vi "read Aux3 from daq 2016.vi"(4 "Descriptions":string[](array[string]), 5 "error in (no error)":errorcluster, 6 "Aux 3 Slope":dbl=1.7339999675750732 format="%.2f", 10 "Array in":refnum<k24>[](array[refnum]), 11 "Sensor Cluster In":T1) -> (12 "Array out":refnum<k24>[](array[refnum]), 13 "Sensor Cluster 2":T1, 14 "Aux3/EC":dbl format="%.2f", 19 "error out":errorcluster)   [LabVIEW 2016]
uses:
  controls/MCC DAQ Readings.ctl
  C:/Cascade-lv16-64/builds/Waterloo Main Program/cascade/data/ULx_LV.dll
  builds/Waterloo Main Program/cascade/data/ULx_LV.dll
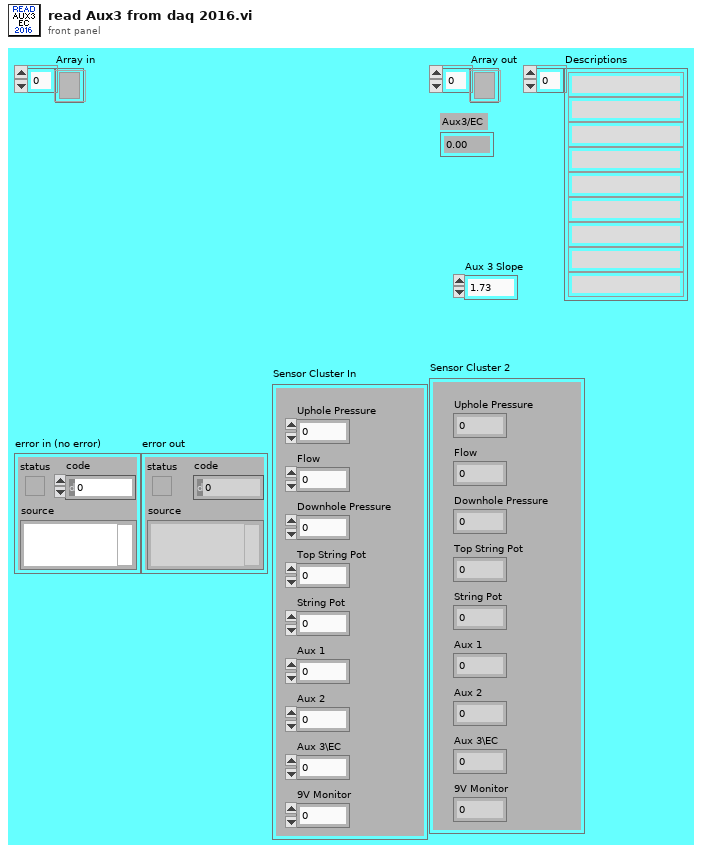
[diagram p1: front panel]
types:
  T1 = typedef "MCC DAQ Readings.ctl" = cluster{"Uphole Pressure":dbl, "Flow":dbl, "Downhole Pressure":dbl, "Top String Pot":dbl, "String Pot":dbl, "Aux 1":dbl, "Aux 2":dbl, "Aux 3\\EC":dbl, "9V Monitor":dbl}
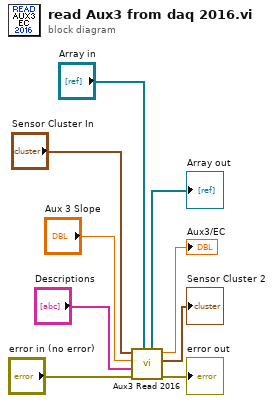
[diagram p0: block diagram]
diagram:
  n1 = call "Aux3 Read 2016.vi"("Array in"="Array in", "error in (no error)"="error in (no error)", "Descriptions"="Descriptions", "Aux3 Slope In"="Aux 3 Slope", "Sensor Cluster"="Sensor Cluster In") -> ("error out"=→"error out":errorcluster, "Sensor Cluster 2"=→"Sensor Cluster 2":T1, "Aux3\\EC Out"=→"Aux3/EC":dbl, "Array out"=→"Array out":refnum<k24>[])  [unwired: 3 in]
